vi "Get SubpanelVI Info.vi"(8 "error in (no error)":errorcluster, 11 "Motions Configuration in":refnum<class "Motions Configuration.lvclass">) -> (0 "error out":errorcluster, 1 "Array of Subpanel VI data":T1[](array[typedef]), 2 "Array of Category string":string[](array[string]), 3 "Motions Configuration out":refnum<class "Motions Configuration.lvclass">)   [LabVIEW 2016, in "Hardware.lvlib" / "Motions.lvlib" / "Motions Configuration.lvclass"]
uses:
  <userlib>/Common Components/Hardware/Abstract System/Motions/Motions Config/Motions Configuration.lvclass
  <userlib>/Configuration Dialog Actor/Methods/Data Retrieved by Lookup Table.ctl
  <userlib>/Configuration Dialog Actor/Configuration.lvclass
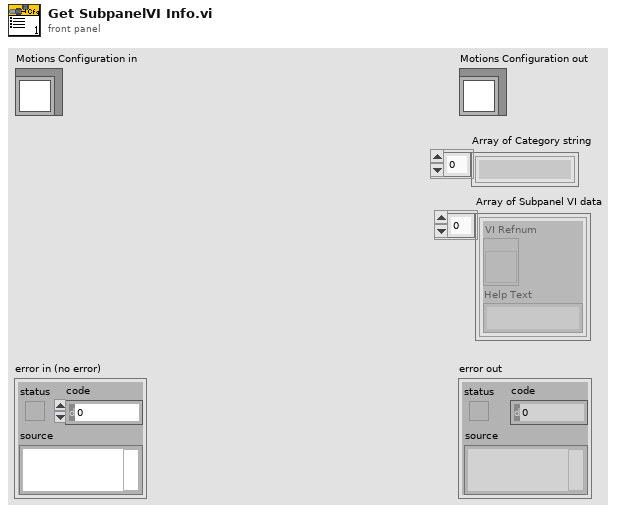
[diagram p1: front panel]
types:
  T1 = typedef "Configuration.lvlib/Configuration.lvclass/Data Retrieved by Lookup Table.ctl" = cluster{"VI Refnum":refnum<vi>, "Help Text":string}
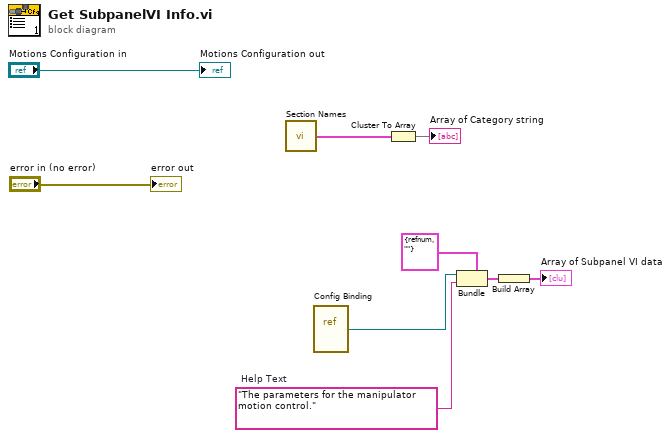
[diagram p0: block diagram]
diagram:
  w3 = "The parameters for the manipulator motion control."  # Help Text
  n1 = call <userlib>:"Section Names.vi"() -> ("Cluster"=w1:cluster{"Motion Settings":string})
  n2 = vi-ref <userlib>:"Config Binding.vi"() -> (w4:refnum<vi>)
  n3 = Cluster To Array(cluster=w1) -> (array=→"Array of Category string":string[])
  n4 = Bundle(cluster=T1 {"VI Refnum"=refnum, "Help Text"=""} ("output cluster"), "VI Refnum"=w4, "Help Text"=w3) -> (w5:T1)
  n5 = Build Array(w5) -> (→"Array of Subpanel VI data":T1[])
  "error out" <- "error in (no error)"
  "Motions Configuration out" <- "Motions Configuration in"
